vi "Maj.vi"(9 "z":u32, 10 "y":u32, 11 "x":u32) -> (3 "Maj":u32)   [LabVIEW 2013, in "NI_SHA-256(2013).lvlib" / "NI_SHA-256.lvclass"]
doc: "Computes the function Maj(x, y, z) as defined in the SHA-2 specification."
uses:
  NI_SHA-256.lvclass
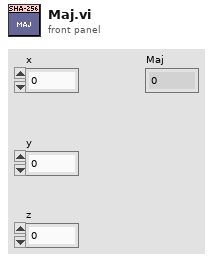
[diagram p1: front panel]
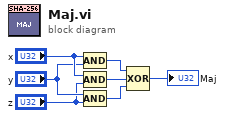
[diagram p0: block diagram]
diagram:
  n1 = Compound Arithmetic op=AND("x", "y") -> (w7:u32)
  n2 = Compound Arithmetic op=AND("x", "z") -> (w6:u32)
  n3 = Compound Arithmetic op=AND("y", "z") -> (w5:u32)
  n4 = Compound Arithmetic op=XOR(w7, w6, w5) -> (→"Maj":u32)
